vi "main.vi"() -> ()   [LabVIEW 2010]
uses:
  common/xcontrols/XImage/XImage/XImage.xctl
  common/classes/ImageCollection/ImageCollection/ImageCollection.lvclass
  section_cluster.ctl
  <vilib>/Utility/file.llb/Write To Spreadsheet File (string).vi
  <vilib>/Utility/file.llb/Write To Spreadsheet File (DBL).vi
panel:
  in  "section index":i32(slide) min=0 max=1000 scale=0.0..9.0
  in  "sections":T1[](array[typedef]) {"stop index" min=1; "start index" min=1}
  in  "initial offset":i32=10 min=1
  in  "button:export":bool
  in  "moving average window size":i32=5
  out "trace":sgl[][](graph)
  in  "button:stop":bool
  in  "XImage":refnum<class "ImageCollection.lvclass">(xcontrol)
  # "LineScanAnalyserDL120829"
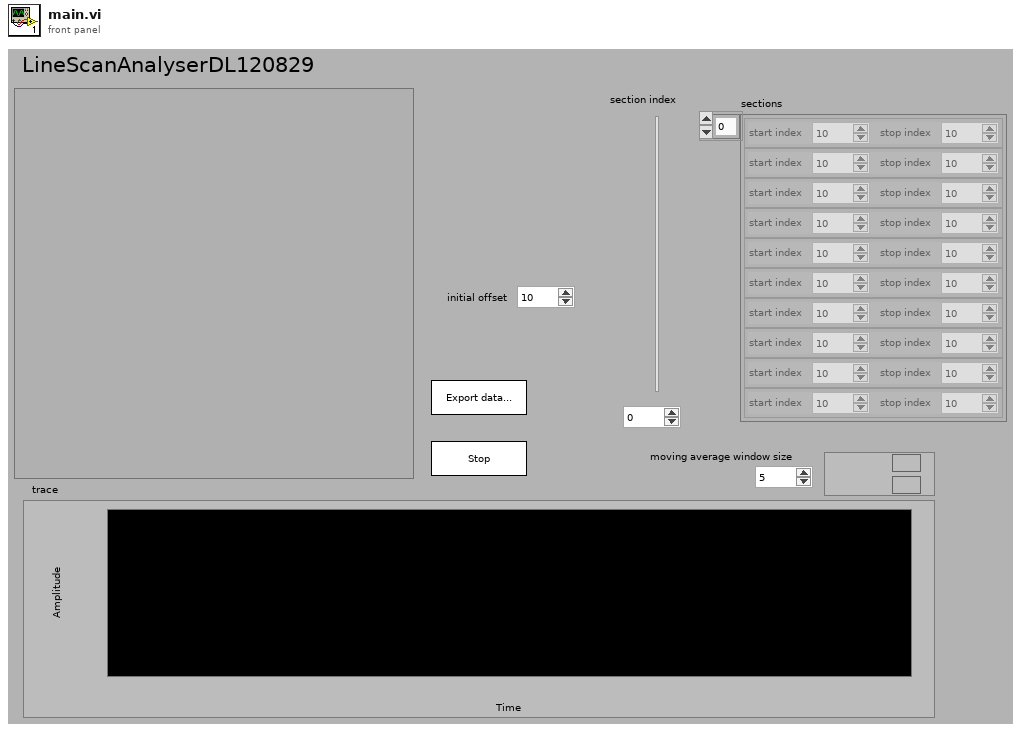
[diagram p1: front panel]
types:
  T1 = typedef "section_cluster.ctl" = cluster{"start index":i32, "stop index":i32}
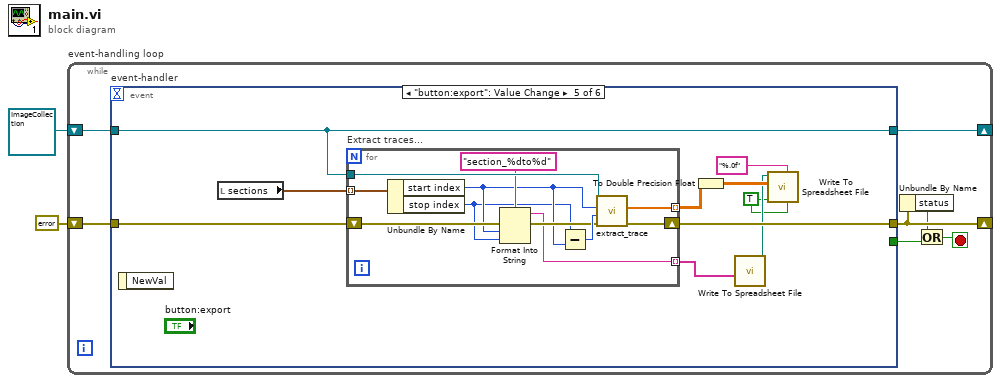
[diagram p0: block diagram]
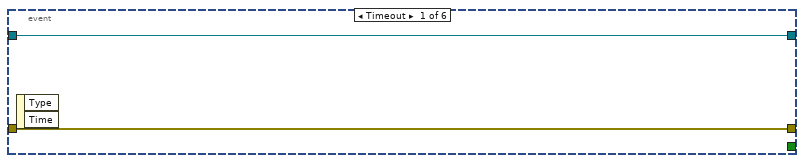
[diagram p2: hidden frame]
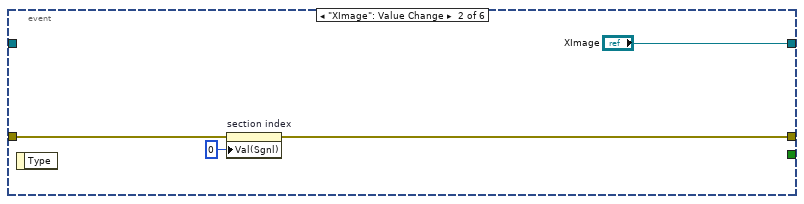
[diagram p3: hidden frame]
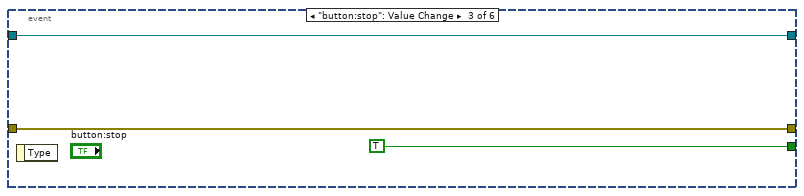
[diagram p4: hidden frame]
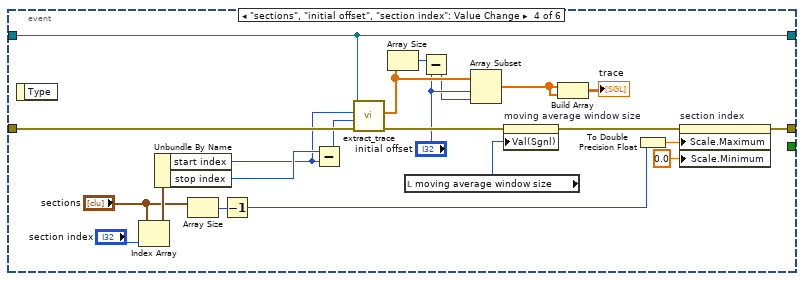
[diagram p5: hidden frame]
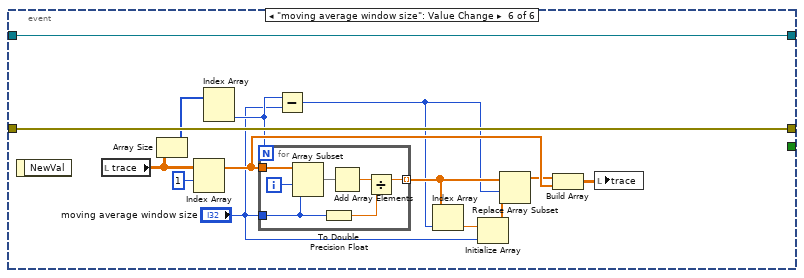
[diagram p6: hidden frame]
diagram:
  n1 = while "event-handling loop" {
    shift-right: [w9] -> _
    shift-left: refnum<class "ImageCollection.lvclass"> refnum ("ImageCollection.lvclass") -> [w8]
    shift-right: [w6] -> _
    shift-left: errorcluster {"status"=FALSE, "code"=0, "source"=""} ("error out") -> [w7]
    stop <- w3 stop-if-true
    n2 = event "event-handler" shown="[4] \"button:export\": Value Change" {
      selector: _ -> [_ _ _ _ _ _]
      dyn-events: _ -> [_ _ _ _ _ _]
      timeout: _ -> [_ _ _ _ _ _]
      tunnel: [w11 "XImage" w18 w36 w46 w75] -> w9
      tunnel: w8 -> [w11 _ w18 w36 w46 w75]
      tunnel: [_ _ TRUE _ _ _] -> w5
      tunnel: w7 -> [w10 w14 w16 w40 w49 w74]
      tunnel: [w10 w13 w16 w22 w48 w74] -> w6
      event Timeout {
        n3 = event-data() -> ()  [unwired: 1 in, 2 out]
      }
      event "XImage": Value Change {
        n4 = event-data() -> ()  [unwired: 1 in, 1 out]
        n5 = property on="section index" class="Slide (strict)"(error in=w14, "Val(Sgnl)"=0 ("Value (Signaling)")) -> (error out=w13:errorcluster)  [unwired: 1 in, 1 out]
      }
      event "button:stop": Value Change {
        n6 = event-data() -> ()  [unwired: 1 in, 1 out]
      }
      event "sections", "initial offset", "section index": Value Change {
        n7 = event-data() -> ()  [unwired: 1 in, 1 out]
        n8 = Index Array(array="sections", index="section index") -> (element=w28:T1)
        n9 = Unbundle By Name(w28) -> ("start index"=w26:i32, "stop index"=w27:i32)
        n10 = Array Size(array="sections") -> (size(s)=w21:i32)
        n11 = Decrement(x=w21) -> (x-1=w20:i32)
        n12 = Subtract(x=w27, y=w26) -> (x-y=w30:i32)
        n13 = call "extract_trace.vi"("error in (no error)"=w40, "sub-pixels"=w30, "start index"=w26, "ImageCollection in"=w36) -> ("error out"=w37:errorcluster, "trace"=w35:sgl[])  [unwired: 6 in]
        n14 = Array Size(array=w35) -> (size(s)=w34:i32)
        n15 = local read "moving average window size"() -> (w38:i32)
        n16 = Subtract(x=w34, y="initial offset") -> (x-y=w32:i32)
        n17 = Array Subset(array=w35, index="initial offset", length=w32) -> (w31:sgl[])
        n18 = property on="moving average window size" class="DigNum (strict)"(error in=w37, "Val(Sgnl)"=w38) -> (error out=w23:errorcluster)  [unwired: 1 in, 1 out]
        n19 = Build Array(w31, w31) -> (→"trace":sgl[][])
        n20 = To Double Precision Float(number=w20) -> (double precision float=w24:dbl)
        n21 = property on="section index" class="Slide (strict)"(error in=w23, "Scale.Maximum"=w24, "Scale.Minimum"=0.0 ("Scale.Range:Minimum")) -> (error out=w22:errorcluster)  [unwired: 1 in, 1 out]
      }
      event "button:export": Value Change {
        w41 = TRUE ("append to file? (new file:F)")
        n22 = event-data() -> ()  [unwired: 1 in, 1 out]
        n23 = local read "sections"() -> (w47:T1[])
        n24 = for "Extract traces..." {
          shift-right: [w61] -> w48
          shift-left: w49 -> [w57]
          tunnel: w47 -> [w60] mode=indexing
          tunnel: w46 -> [w59]
          tunnel: [w55] -> w45 mode=indexing
          tunnel: [w54] -> w43 mode=indexing
          n25 = Unbundle By Name(w60) -> ("start index"=w52:i32, "stop index"=w51:i32)
          n26 = Format Into String(format string="section_%dto%d" ("initial string"), error in=w57, w52, w51) -> (resulting string=w54:string, error out=w56:errorcluster)  [unwired: 1 in]
          n27 = Subtract(x=w51, y=w52) -> (x-y=w58:i32)
          n28 = call "extract_trace.vi"("error in (no error)"=w56, "sub-pixels"=w58, "start index"=w52, "ImageCollection in"=w59) -> ("error out"=w61:errorcluster, "trace"=w55:sgl[])  [unwired: 6 in]
        }
        n29 = To Double Precision Float(number=w45) -> (double precision float=w44:dbl[][])
        n30 = call-poly <vilib>:"Write To Spreadsheet File.vi"("1D data"=w43) -> ("new file path (Not A Path if cancelled)"=w42:path)  [unwired: 7 in]
        n31 = call-poly <vilib>:"Write To Spreadsheet File.vi"("transpose? (no:F)"=w41, "format (%.3f)"="%.0f", "append to file? (new file:F)"=w41, "2D data"=w44, "file path (dialog if empty)"=w42) -> ()  [unwired: 3 in, 1 out]
      }
      event "moving average window size": Value Change {
        n32 = event-data() -> ()  [unwired: 1 in, 1 out]
        n33 = local read "trace"() -> (w71:sgl[][])
        n34 = Array Size(array=w71) -> (size(s)=w70:i32[])
        n35 = Index Array(array=w71, index (row)=1) -> (element=w69:sgl[])  [unwired: 1 in]
        n36 = Index Array(array=w70) -> (element #2=w67:i32)  [unwired: 2 in, 1 out]
        n37 = for {
          N: w67 -> [_]
          tunnel: w69 -> [w82]
          tunnel: "moving average window size" -> [w77]
          tunnel: [w78] -> w66 mode=indexing
          i -> [w81]
          n38 = Array Subset(array=w82, index=w81, length=w77) -> (w80:sgl[])
          n39 = To Double Precision Float(number=w77) -> (double precision float=w76:dbl)
          n40 = Add Array Elements(numeric array=w80) -> (sum=w79:sgl)
          n41 = Divide(x=w79, y=w76) -> (x/y=w78:dbl)
        }
        n42 = Subtract(x=w67, y="moving average window size") -> (x-y=w65:i32)
        n43 = Index Array(array=w66, index=w65) -> (element=w64:dbl)
        n44 = Initialize Array(w64, "moving average window size") -> (w62:dbl[])
        n45 = Replace Array Subset(array=w66, new element=w62, index=w65) -> (w68:dbl[])
        n46 = Build Array(w68, w69) -> (w72:dbl[][])
        n47 = local write "trace"(w72) -> ()
      }
    }
    n48 = Unbundle By Name(w6) -> ("status"=w4:bool)
    n49 = Or(x=w4, y=w5) -> (x .or. y?=w3:bool)
  }
